vi "Datatype Assert Helper.vi"(11 "JSON":string) -> (0 "error out":errorcluster, 2 "JSONText (Assert)":string, 3 "JKIJSON (Assert)":string)   [LabVIEW 2018, in "JSON to LVConstant Test.lvlib"]
uses:
  JSON to LVConstant Test.lvlib
  825a1b9b-bd0c-4d13-827c-a2d730ac4f1d.vi
  0098da80-d38a-4bc8-be04-a50e7c1996e8.vi
  <vilib>/JDP Science/JSONtext/JSON text to Variant.vi
  <vilib>/JDP Science/JSONtext/Variant to JSON Text.vi
  <vilib>/JDP Science/JSONtext/LVClass Serializer/JSONtext LVClass Serializer.lvclass
  <vilib>/addons/_JKI.lib/Serialization/JSON/JKI JSON Serialization.lvlib
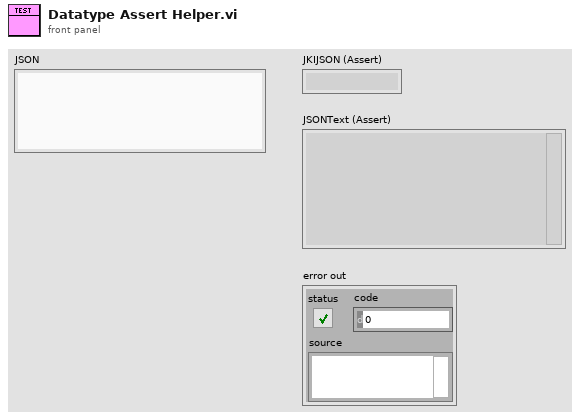
[diagram p1: front panel]
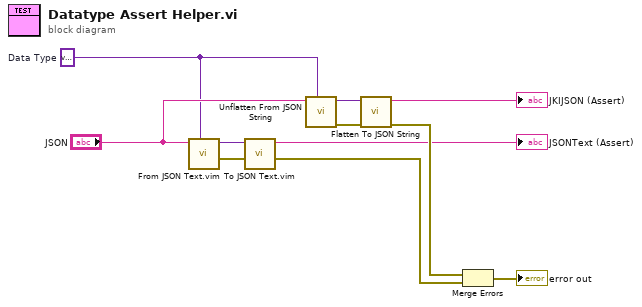
[diagram p0: block diagram]
diagram:
  w10 = variant  # Data Type
  n1 = call "From JSON Text.vim"("Data Type and Default Value"=w10, "JSON"="JSON") -> ("error out"=w9:errorcluster, "Data out"=w3:variant)  [unwired: 8 in]
  n2 = call "To JSON Text.vim"("error in (no error)"=w9, "Anything"=w3) -> ("error out"=w4:errorcluster, "<JSON>"=→"JSONText (Assert)":string)  [unwired: 8 in]
  n3 = call <vilib>:"Unflatten From JSON String.vi"("Type and Defaults"=w10, "JSON String"="JSON") -> ("error out"=w7:errorcluster, "Variant"=w6:variant)  [unwired: 8 in]
  n4 = call <vilib>:"Flatten To JSON String.vi"("error in (no error)"=w7, "Variant"=w6) -> ("error out"=w5:errorcluster, "JSON String"=→"JKIJSON (Assert)":string)  [unwired: 8 in]
  n5 = Merge Errors(w5, w4) -> (→"error out":errorcluster)
